vi "line extraction.vi"(2 "error in (no error)":errorcluster, 3 "Image":T1) -> (0 "error out":errorcluster, 1 "Image Dst Out":T1)   [LabVIEW 2012]
uses:
  <vilib>/vision/Image Controls.llb/IMAQ Image.ctl
  E:/Adam N/Q Summer '12 Image Processing/Type Defs/Images.ctl
  <vilib>/vision/NI_Vision_Development_Module.lvlib
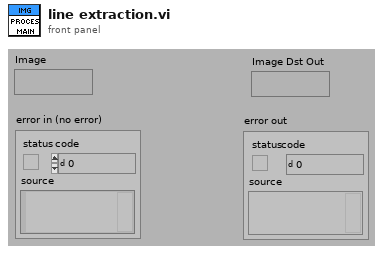
[diagram p1: front panel]
types:
  T1 = typedef "IMAQ Image.ctl" = refnum<image>
  T2 = cluster{"Measurement Parameter":i32, "Range Lower Value":dbl, "Range Upper Value":dbl, "Range":bool, "Measurement Type":bool}[]
  T3 = enum32{"AutoM", "Close", "Dilate", "Erode", "Gradient", "Gradient out", "Gradient in", "Hit miss", "Open", "PClose", "POpen", "Thick", "Thin"}
  T4 = enum32{"Linear", "Log", "Exp", "Square", "Square root", "Power X", "Power 1/X"}
  T5 = typedef "Images.ctl" = cluster{"Camera Image":T1, "Processed Image":T1, "Box Image":T1, "Binary Image":T1}
  T6 = cluster{"Blue Alpha":sgl, "Hue Alpha":sgl, "Lum Alpha":sgl}
  T7 = typedef "Image Type" = u32
  T8 = cluster{"Camera Image":T1, "Processed Image":T1, "Box Image":T1}
  T9 = cluster{"Hue Threshold":sgl, "Blue Threshold":sgl, "Lum Threshold":sgl}
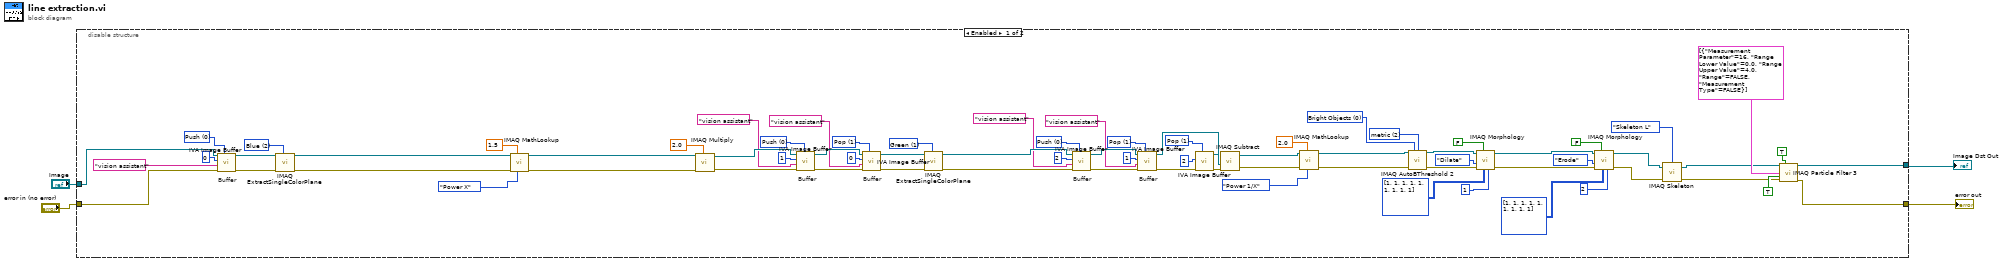
[diagram p0: block diagram]
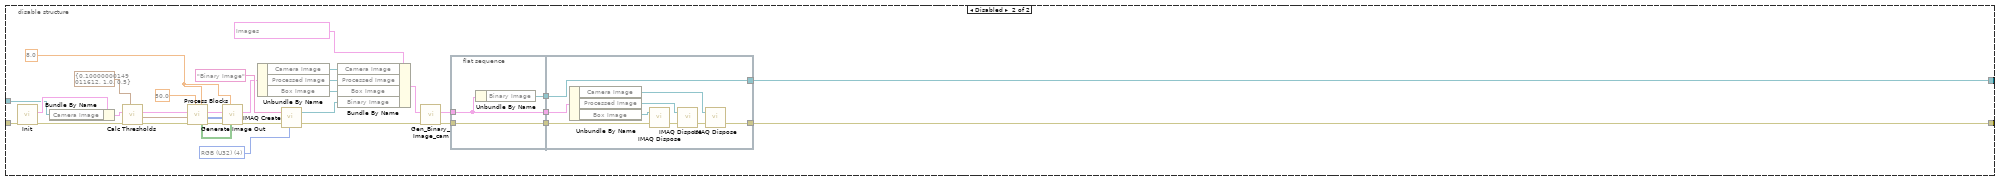
[diagram p2: hidden frame]
diagram:
  n1 = disable-structure shown="Enabled" {
    disable-tunnel: [w5 w85] -> w1
    disable-tunnel: [w6 w79] -> w4
    disable-tunnel: "Image" -> [w16 w109]
    disable-tunnel: "error in (no error)" -> [w15 w111]
    frame Enabled {
      w28 = 2 items=["clustering", "entropy", "metric", "moments", "inter-class variance"] ("Method")
      w29 = u32 0 items=["Bright Objects", "Dark Objects"] ("Look For")
      w41 = u16 1 items=["Push", "Pop", "Reset"] ("Function")
      w44 = u16 1 items=["Push", "Pop", "Reset"] ("Function")
      w49 = u16 0 items=["Push", "Pop", "Reset"] ("Function")
      w54 = 1 items=["Red", "Green", "Blue", "Hue", "Saturation", "Luminance", "Value", "Intensity"] ("Color Plane")
      w57 = u16 1 items=["Push", "Pop", "Reset"] ("Function")
      w62 = u16 0 items=["Push", "Pop", "Reset"] ("Function")
      w74 = 2 items=["Red", "Green", "Blue", "Hue", "Saturation", "Luminance", "Value", "Intensity"] ("Color Plane")
      w77 = u16 0 items=["Push", "Pop", "Reset"] ("Function")
      # "Buffer"
      # "Buffer"
      # "Buffer"
      # "Buffer"
      # "Buffer"
      n2 = call <vilib>:"IVA Image Buffer.vi"("Function"=w77, "error in (no error)"=w15, "Prefix"="vision assistant", "Buffer #"=0, "Image In"=w16) -> ("error out"=w78:errorcluster, "Image Out"=w73:T1)  [unwired: 5 out]
      n3 = call "IMAQ ExtractSingleColorPlane"("Color Plane"=w74, "error in (no error)"=w78, "Image Src"=w73) -> ("error out"=w72:errorcluster, "Image Dst Out"=w69:T1)  [unwired: 1 in, 6 out]
      n4 = call "IMAQ MathLookup"("Operator"=T4."Power X", "X Value"=sgl 1.5, "error in (no error)"=w72, "Image Src"=w69) -> ("error out"=w68:errorcluster, "Image Dst Out"=w66:T1)  [unwired: 3 in, 3 out]
      n5 = call "IMAQ Multiply"("Image Src A"=w66, "Constant"=sgl 2.0, "error in (no error)"=w68) -> ("Image Dst Out"=w64:T1, "error out"=w65:errorcluster)  [unwired: 2 in, 2 out]
      n6 = call <vilib>:"IVA Image Buffer.vi"("Function"=w62, "error in (no error)"=w65, "Prefix"="vision assistant", "Buffer #"=1, "Image In"=w64) -> ("error out"=w63:errorcluster, "Image Out"=w59:T1)  [unwired: 5 out]
      n7 = call <vilib>:"IVA Image Buffer.vi"("Function"=w57, "error in (no error)"=w63, "Prefix"="vision assistant", "Buffer #"=0, "Image In"=w59) -> ("error out"=w58:errorcluster, "Image Out"=w53:T1)  [unwired: 5 out]
      n8 = call "IMAQ ExtractSingleColorPlane"("Color Plane"=w54, "error in (no error)"=w58, "Image Src"=w53) -> ("error out"=w52:errorcluster, "Image Dst Out"=w51:T1)  [unwired: 1 in, 6 out]
      n9 = call <vilib>:"IVA Image Buffer.vi"("Function"=w49, "error in (no error)"=w52, "Prefix"="vision assistant", "Buffer #"=2, "Image In"=w51) -> ("error out"=w50:errorcluster, "Image Out"=w46:T1)  [unwired: 5 out]
      n10 = call <vilib>:"IVA Image Buffer.vi"("Function"=w44, "error in (no error)"=w50, "Prefix"="vision assistant", "Buffer #"=1, "Image In"=w46) -> ("error out"=w45:errorcluster, "Image Out"=w37:T1)  [unwired: 5 out]
      n11 = call <vilib>:"IVA Image Buffer.vi"("Function"=w41, "error in (no error)"=w45, "Buffer #"=2) -> ("error out"=w38:errorcluster, "Image Out"=w39:T1)  [unwired: 2 in, 5 out]
      n12 = call "IMAQ Subtract"("Image Src A"=w37, "Image Src B"=w39, "error in (no error)"=w38) -> ("Image Dst Out"=w33:T1, "error out"=w36:errorcluster)  [unwired: 2 in, 2 out]
      n13 = call "IMAQ MathLookup"("Operator"=T4."Power 1/X", "X Value"=sgl 2.0, "error in (no error)"=w36, "Image Src"=w33) -> ("error out"=w32:errorcluster, "Image Dst Out"=w31:T1)  [unwired: 3 in, 3 out]
      n14 = call "IMAQ AutoBThreshold 2"("Image Src"=w31, "Look For (Bright Objects)"=w29, "Method (clustering)"=w28, "error in (no error)"=w32) -> ("Image Dst Out"=w23:T1, "error out"=w30:errorcluster)  [unwired: 4 in, 6 out]
      n15 = call "IMAQ Morphology"("Number of iterations (1)"=1, "Structuring Element"=i32[][] [[1, 1, 1], [1, 1, 1], [1, 1, 1]], "Square/Hexa (Square)"=FALSE, "error in (no error)"=w30, "Operation"=T3."Dilate", "Image Src"=w23) -> ("error out"=w22:errorcluster, "Image Dst Out"=w17:T1)  [unwired: 1 in, 3 out]
      n16 = call "IMAQ Morphology"("Number of iterations (1)"=2, "Structuring Element"=i32[][] [[1, 1, 1], [1, 1, 1], [1, 1, 1]], "Square/Hexa (Square)"=FALSE, "error in (no error)"=w22, "Operation"=T3."Erode", "Image Src"=w17) -> ("error out"=w12:errorcluster, "Image Dst Out"=w14:T1)  [unwired: 1 in, 3 out]
      n17 = call "IMAQ Skeleton"("error in (no error)"=w12, "Image Src"=w14, "Mode"=enum32{"Skeleton L", "Skeleton M", "Skiz"}."Skeleton L") -> ("error out"=w7:errorcluster, "Image Dst Out"=w8:T1)  [unwired: 3 in]
      n18 = call "IMAQ Particle Filter 3"("Image Src"=w8, "Connectivity 4/8 (8)"=TRUE, "Selection Values"=T2 [{"Measurement Parameter"=16, "Range Lower Value"=0.0, "Range Upper Value"=4.0, "Range"=FALSE, "Measurement Type"=FALSE}], "Keep/Remove Particles (F)"=TRUE ("Keep/Remove Particles"), "error in (no error)"=w7) -> ("Image Dst Out"=w6:T1, "error out"=w5:errorcluster)  [unwired: 4 in, 5 out]
    }
    frame Disabled {
      w95 = T7 4 items=["Grayscale (U8)", "Grayscale (I16)", "Grayscale (SGL)", "Complex (CSG)", "RGB (U32)", "HSL (U32)", "RGB (U64)", "Grayscale (U16)"] ("Image Type")
      w97 = 8.0 ("Block Size")
      n19 = call "Init.vi"("error in (no error)"=w111) -> ("error out"=w108:errorcluster, "Images Out"=w110:T8)  [unwired: 9 in]
      n20 = Bundle By Name(cluster=w110, "Camera Image"=w109) -> (w107:T8)
      n21 = call "Calc Thresholds.vi"("Alphas"=T6 {"Blue Alpha"=0.1, "Hue Alpha"=1.0, "Lum Alpha"=0.5}, "error in (no error)"=w108, "Images In"=w107) -> ("error out"=w105:errorcluster, "Thresholds"=w104:T9, "Images Out"=w103:T8)  [unwired: 4 in, 2 out]
      n22 = call "Process Blocks.vi"("Block Size"=w97, "Range"=50.0, "error in (no error)"=w105, "Thresholds"=w104, "Images In"=w103) -> ("error out"=w99:errorcluster, "Image Array"=w101:u32[][], "Images Out"=w100:T8, "Occupied Array"=w98:bool[][])  [unwired: 3 in]
      n23 = call "Generate Image Out.vi"("Occupied Array"=w98, "Block Size"=w97, "error in (no error)"=w99, "Image Array In"=w101, "Images In"=w100) -> ("error out"=w89:errorcluster, "Images Out"=w88:T8)  [unwired: 5 in]
      n24 = Unbundle By Name(w88) -> ("Camera Image"=w92:T1, "Processed Image"=w91:T1, "Box Image"=w90:T1)
      n25 = call "IMAQ Create"("Image Name"="Binary Image", "Image Type"=w95, "error in (no error)"=w89) -> ("New Image"=w93:T1, "error out"=w84:errorcluster)  [unwired: 2 in]
      n26 = Bundle By Name(cluster=T5 {"Camera Image"=refnum, "Processed Image"=refnum, "Box Image"=refnum, "Binary Image"=refnum} ("Images"), "Camera Image"=w92, "Processed Image"=w91, "Box Image"=w90, "Binary Image"=w93) -> (w83:T5)
      n27 = call "Gen_Binary_Image_cam.vi"("Images In"=w83, "error in (no error)"=w84) -> ("Images Out"=w82:T5, "error out"=w81:errorcluster)  [unwired: 7 in]
      n28 = flat-sequence {
        tunnel: w81 -> [w113]
        tunnel: [w114] -> w87
        tunnel: [w113] -> w86
        tunnel: w82 -> [w112]
        tunnel: [w112] -> w80
        tunnel: [w123] -> w79
        tunnel: w87 -> [w123]
        tunnel: w86 -> [w122]
        tunnel: [w119] -> w85
        tunnel: w80 -> [w118]
        frame #0 {
          n29 = Unbundle By Name(w112) -> ("Binary Image"=w114:T1)
        }
        frame #1 {
          n30 = Unbundle By Name(w118) -> ("Camera Image"=w115:T1, "Processed Image"=w116:T1, "Box Image"=w117:T1)
          n31 = call "IMAQ Dispose"("Image"=w117, "error in (no error)"=w122) -> ("error out"=w121:errorcluster)  [unwired: 4 in]
          n32 = call "IMAQ Dispose"("Image"=w116, "error in (no error)"=w121) -> ("error out"=w120:errorcluster)  [unwired: 4 in]
          n33 = call "IMAQ Dispose"("Image"=w115, "error in (no error)"=w120) -> ("error out"=w119:errorcluster)  [unwired: 4 in]
        }
      }
    }
  }
  "error out" <- w1
  "Image Dst Out" <- w4
